vi "Variably-sized Cluster.vi"   [LabVIEW 2020, in "Memory Manager Tests.lvlib" / "Malleable Type Tests.lvclass"]
uses:
  Malleable Type Tests.lvclass
  Source/Classes/Pointer/Pointer.lvclass
  ba8e9364-ef61-494a-a3e2-0ca29be4377a.vi
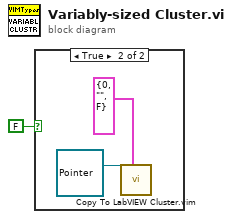
[diagram p0: block diagram]
diagram:
  n1 = case shown="True" FALSE {
    frame False {
    }
    frame True {
      n2 = call "Copy To LabVIEW Cluster.vim"("Type"=cluster{i32, string, bool} {0, "", FALSE}, "Pointer in"=refnum<class "Pointer.lvclass"> refnum) -> ()  [unwired: 7 in, 3 out]
    }
  }
